vi "User Interface Event Handler.vi"() -> ()   [LabVIEW 2013]
panel:
  out "a+b":dbl
  in  "b":dbl
  in  "a":dbl
  in  "stop":bool
  in  "add":bool
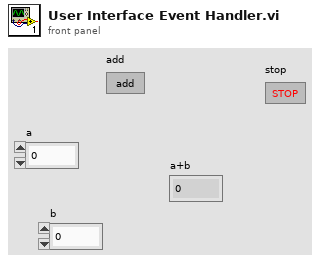
[diagram p1: front panel]
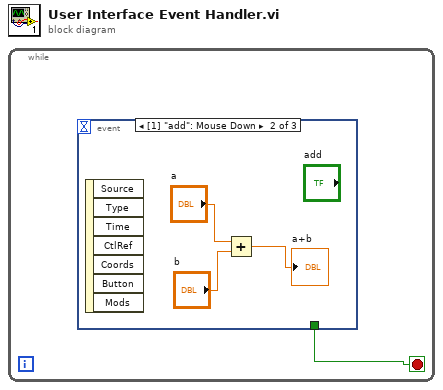
[diagram p0: block diagram]
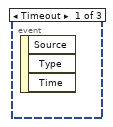
[diagram p2: hidden frame]
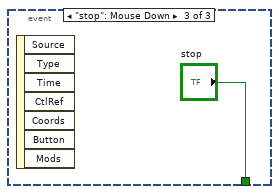
[diagram p3: hidden frame]
diagram:
  n1 = while {
    stop <- w1 stop-if-true
    n2 = event shown="[1] \"add\": Mouse Down" {
      selector: _ -> [_ _ _]
      dyn-events: _ -> [_ _ _]
      timeout: _ -> [_ _ _]
      tunnel: [_ _ "stop"] -> w1
      event Timeout {
        n3 = event-data() -> ()  [unwired: 1 in, 3 out]
      }
      event "add": Mouse Down {
        n4 = event-data() -> ()  [unwired: 1 in, 7 out]
        n5 = Add(x="a", y="b") -> (x+y=→"a+b":dbl)
      }
      event "stop": Mouse Down {
        n6 = event-data() -> ()  [unwired: 1 in, 7 out]
      }
    }
  }
